vi "Minus.vi"(7 "Abs?":bool, 9 "Readable B":refnum<class "Readable.lvclass">, 10 "Readable A":refnum<class "Readable.lvclass">) -> (1 "error out":errorcluster, 2 "Minus.lvclass out":refnum<class "Minus.lvclass">)   [LabVIEW 2009, in "Minus.lvclass"]
uses:
  Minus.lvclass
  Readable/Readable.lvclass
  Minus.lvclass/Minus.ctl
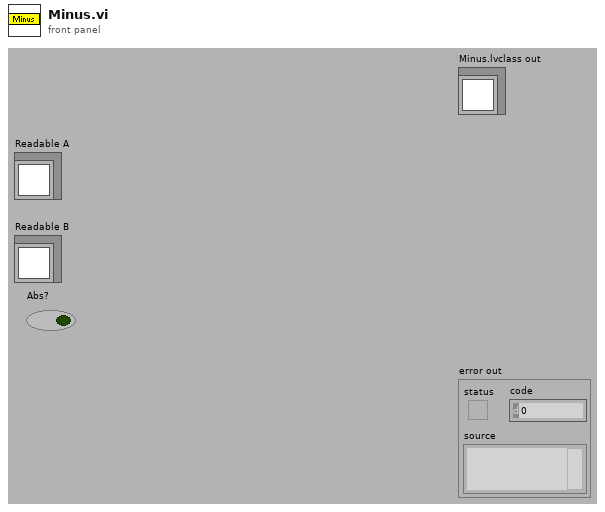
[diagram p1: front panel]
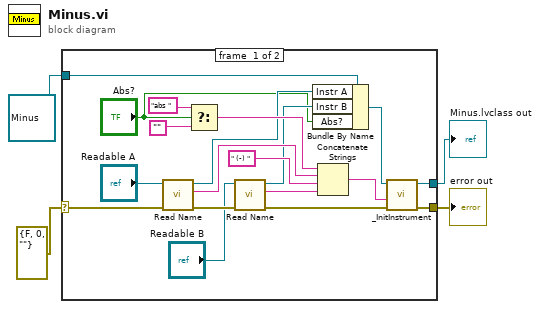
[diagram p0: block diagram]
diagram:
  n1 = case shown="No Error" errorcluster {"status"=FALSE, "code"=0, "source"=""} ("error in (no error)") {
    selector: errorcluster {"status"=FALSE, "code"=0, "source"=""} ("error in (no error)") -> [w10 w24]
    tunnel: [w13 w24] -> w3
    tunnel: [w7 w25] -> w1
    tunnel: refnum<class "Minus.lvclass"> refnum ("Minus.lvclass in") -> [w6 w25]
    frame #0 {
      n2 = call-dynamic "Read Name.vi"("error in (no error)"=w10, "Instrument.lvclass in"="Readable A") -> ("error out"=w15:errorcluster, "Name"=w18:string, "Instrument.lvclass out"=w16:refnum<class "Readable.lvclass">)  [unwired: 7 out]
      n3 = Select(t="abs ", s="Abs?", f="") -> (s? t:f=w23:string)
      n4 = call-dynamic "Read Name.vi"("error in (no error)"=w15, "Instrument.lvclass in"="Readable B") -> ("error out"=w14:errorcluster, "Name"=w20:string, "Instrument.lvclass out"=w17:refnum<class "Readable.lvclass">)  [unwired: 7 out]
      n5 = Bundle By Name(cluster=w6, "Instr A"=w16, "Instr B"=w17, "Abs?"="Abs?") -> (w5:refnum<class "Minus.lvclass">)
      n6 = Concatenate Strings(w23, w18, " (-) ", w20) -> (w8:string)
      n7 = call-dynamic "_InitInstrument.vi"("error in (no error)"=w14, "Name"=w8, "Instrument in"=w5) -> ("error out"=w13:errorcluster, "Instrument out"=w7:refnum<class "Minus.lvclass">)  [unwired: 3 in, 4 out]
    }
    frame #1 {
    }
  }
  "error out" <- w3
  "Minus.lvclass out" <- w1
